vi "I16 Array To SGL Array.vi"(0 "I16 Array":i16[](array[numeric])=[-13107, 17142, 3072, 17799, -30310, 17559] format="%04x") -> (1 "元素0":sgl, 2 "SGL Array":sgl[](array[numeric]) format="%.3f")   [LabVIEW 2018]
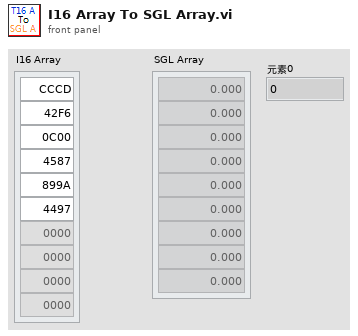
[diagram p1: front panel]
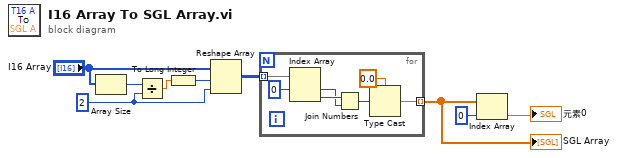
[diagram p0: block diagram]
diagram:
  w4 = 2 ("维数大小")
  n1 = Array Size(array="I16 Array") -> (size(s)=w7:i32)
  n2 = Divide(x=w7, y=w4) -> (x/y=w6:dbl)
  n3 = To Long Integer(number=w6) -> (32bit integer=w5:i32)
  n4 = Reshape Array("I16 Array", w5, w4) -> (w9:i16[][])
  n5 = for {
    tunnel: w9 -> [w16] mode=indexing
    tunnel: [w11] -> w2 mode=indexing
    n6 = Index Array(array=w16, index #1=0 ("索引")) -> (element #1=w13:i16, element #2=w14:i16)  [unwired: 1 in]
    n7 = Join Numbers(hi=w14, lo=w13) -> ((hi.lo)=w12:u32)
    n8 = Type Cast(type=sgl 0.0, x=w12) -> (*(type *) &x=w11:sgl)
  }
  "SGL Array" <- w2
  n9 = Index Array(array=w2, index=0 ("索引")) -> (element=→"元素0":sgl)
